vi "ProcessName.vi"() -> (1 "process name":string="EmsaFpgaBitfileManager")   [LabVIEW 2017, in "EmsaFPGABitfileManager.lvlib"]
uses:
  <vilib>/addons/InsightCM/Devices/Shared/Emsa/EmsaFPGABifileManager/EmsaFPGABitfileManager.lvlib
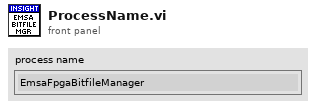
[diagram p1: front panel]
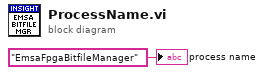
[diagram p0: block diagram]
diagram:
  "process name" <- "EmsaFpgaBitfileManager" ("ProcessName")
